vi "config UI.vi"() -> ()   [LabVIEW 2017, in "WaveformAcq editor node.lvclass"]
doc: "All child modules share this same UI. The UI allows for the configuration of Channels, Parameters, and Error Handling."
uses:
  WaveformAcq editor node.lvclass
  <vilib>/NI/Configuration Framework/Node/NodeRef.ctl
  <vilib>/NI/Configuration Framework/Node/NISE_CEF_Node.lvclass
  <vilib>/NI/AMC/Message Queue.ctl
  <vilib>/NI/AMC/Message.ctl
  <vilib>/NI/Tools/Keyed Array/KeyedArray.ctl
  <vilib>/NI/Configuration Framework/Node/UserEventRef.ctl
  <vilib>/NI/Configuration Framework/Controls/EventCluster.ctl
  <vilib>/NI/DCAF/Tag Editor Core/control module/configuration/error classification setting.ctl
  <vilib>/NI/Tag Bus Module Framework/runtime/error classification.ctl
  <vilib>/NI/Configuration Framework/Node/RefreshUIEvent.ctl
  <vilib>/NI/Configuration Framework/Node/CacheState.ctl
  <vilib>/NI/Configuration Framework/Node/StopEvent.ctl
  <vilib>/NI/Configuration Framework/Node/NodeChangeEvent.ctl
  <vilib>/NI/DCAF/Tag Editor Core/Table API/Available Tag Menu/channel action event.ctl
  <vilib>/NI/DCAF/Tag Editor Core/Table API/Available Tag Menu/dialog output action.ctl
  <vilib>/NI/Tag Bus Module Framework/channel/TBM channel.lvclass
  <vilib>/NI/Tag Bus/tag/tag descriptor.lvclass
  <vilib>/NI/DCAF/Tag Editor Core/Table API/Table Manager/Call Back Ref Type Def.ctl
  <vilib>/NI/DCAF/Tag Editor Core/Configuration Editor/Classes/Engine Parent/Engine Parent Editor Node.lvclass
  <vilib>/NI/DCAF/Tag Editor Core/Configuration Editor/Classes/Module editor node/module editor node.lvclass
  C:/Program Files (x86)/National Instruments/LabVIEW 2017/vi.lib/NI/Configuration Framework/serializable node/NISE_CEF_serializable node.lvclass
  <vilib>/NI/DCAF/Tag Editor Core/Table API/Table Manager/references.ctl
  <vilib>/NI/DCAF/Tag Editor Core/Table API/Table Manager/Menu Definition.ctl
  <vilib>/NI/DCAF/Tag Editor Core/Table API/Table Manager/Menu Options.ctl
  <vilib>/NI/DCAF/Tag Editor Core/control module/configuration/control module configuration.lvclass
  C:/Program Files (x86)/National Instruments/LabVIEW 2017/vi.lib/NI/Configuration Framework/serializable configuration/NISE_CEF_serializable configuration.lvclass
  module/configuration/WaveformAcq configuration.lvclass
  C:/Program Files (x86)/National Instruments/LabVIEW 2017/vi.lib/NI/DCAF/Tag Editor Core/control module/configuration/control module configuration.lvclass
  C:/Program Files (x86)/National Instruments/LabVIEW 2017/vi.lib/NI/Tag Bus Module Framework/module configuration/TBM module configuration.lvclass
  module/configuration/WaveformAcq configuration.lvclass/WaveformAcq configuration.ctl
  <vilib>/NI/DCAF/Tag Editor Core/control module/configuration/control module configuration.lvclass/control module configuration.ctl
  <vilib>/NI/Configuration Framework/serializable configuration/NISE_CEF_serializable configuration.lvclass/NISE_CEF_serializable configuration.ctl
  <vilib>/NI/Tag Bus Module Framework/channel/channel classification.ctl
  <vilib>/NI/DCAF/Tag Editor Core/control module/configuration/Write error classifications.vi
  <vilib>/NI/Tag Bus Module Framework/module configuration/TBM module configuration.lvclass
  <vilib>/NI/DCAF/Tag Editor Core/Configuration Editor/Classes/Module editor node/Read Module Configuration.vi
  <vilib>/Utility/LVClass/Get LV Class Name.vi
  <vilib>/NI/Configuration Framework/error generator/NISE_error generator.vi
  <vilib>/NI/DCAF/Tag Editor Core/Configuration Editor/Classes/Module editor node/Write Module Configuration.vi
  <vilib>/NI/Configuration Framework/serializable configuration/NISE_CEF_serializable configuration.lvclass
  <vilib>/NI/DCAF/Tag Editor Core/Table API/Listbox/Multi Column Listbox.lvclass
  <vilib>/NI/Configuration Framework/NISE_CEF_TreeControl.lvlib
  <vilib>/NI/DCAF/Tag Editor Core/Table API/Table Manager.lvlib
  <vilib>/NI/DCAF UI Toolkit/Controls/DCAF UI Elements.lvlib
  <vilib>/NI/Tools/Keyed Array/Tools_KeyedArray.lvlib
  <vilib>/NI/AMC/AMC.lvlib
  <vilib>/NI/DCAF/Tag Editor Core/Table API/Table Manager/Table Manager.lvclass
  <vilib>/NI/DCAF/Tag Editor Core/control module/editor node/control module editor.lvclass
  <vilib>/NI/Tag Bus Module Framework/runtime/TBM module execution interface.lvclass
panel:
  in  "Enum":i32
  in  "user event out":refnum<user-event>
  in  "Top Level Tab Control":T1(tab)
  in  "Channels Listbox":i32(listbox)
  in  "mapall":bool
  in  "mapwriters":bool
  in  "Parameters Listbox":i32(listbox)
  in  "Order":string[](array[string])
  in  "error classifications":T2[](array[typedef])
  in  "node change":T4
  in  "stop event":T5
  in  "cache state":T6
  in  "refresh UI":T7
  in  "user event":T8
  in  "main queue":T9
  in  "node ref":T10
  # "(Single-Click to Edit)"
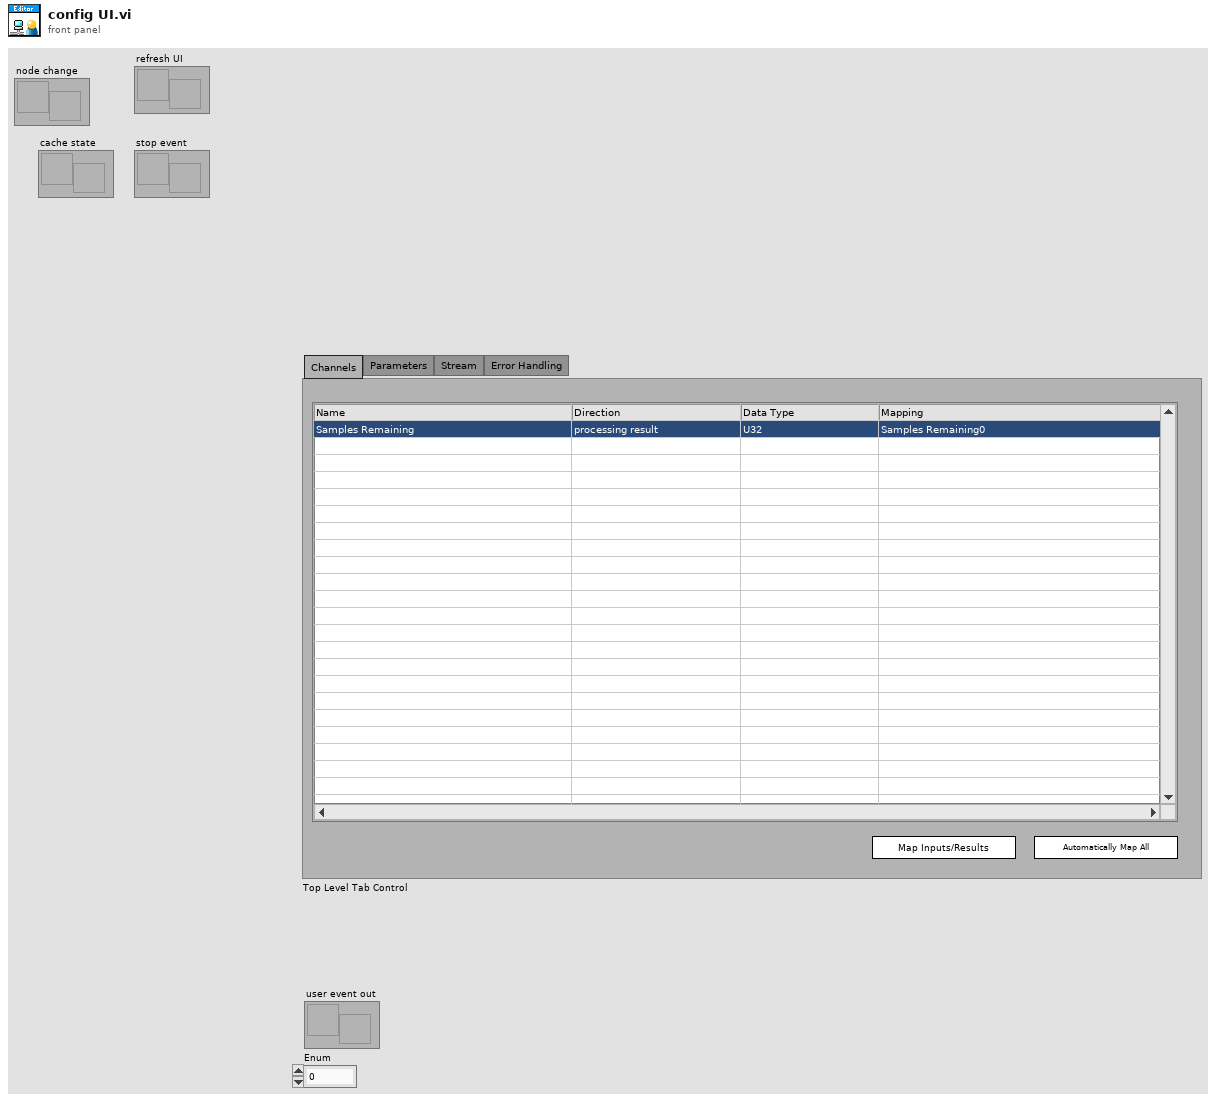
[diagram p1: front panel]
types:
  T1 = enum32{"Channels", "Parameters", "Stream", "Error Handling"}
  T2 = typedef "control module configuration.lvclass/error classification setting.ctl" = cluster{"code":i32, "error classification":T3}
  T3 = typedef "TBM module execution interface.lvclass/error classification.ctl" = enum16{"unknown", "none", "trivial", "recoverable", "critical"}
  T4 = typedef "NISE_CEF_Node.lvclass/NodeChangeEvent.ctl" = refnum<user-event>
  T5 = typedef "NISE_CEF_Node.lvclass/StopEvent.ctl" = refnum<user-event>
  T6 = typedef "NISE_CEF_Node.lvclass/CacheState.ctl" = refnum<user-event>
  T7 = typedef "NISE_CEF_Node.lvclass/RefreshUIEvent.ctl" = refnum<user-event>
  T8 = typedef "NISE_CEF_Node.lvclass/UserEventRef.ctl" = refnum<user-event>
  T9 = typedef "AMC.lvlib/Message Queue.ctl" = refnum<queue>
  T10 = typedef "NISE_CEF_Node.lvclass/NodeRef.ctl" = refnum<data-value>
  T11 = typedef "Table Manager.lvlib/Table Manager.lvclass/Menu Definition.ctl" = cluster{"Menu Name":string, "Menu Options":T12}
  T12 = typedef "Table Manager.lvlib/Table Manager.lvclass/Menu Options.ctl" = enum16{"Always Show", "Show When Used", "Show When Empty"}
  T13 = typedef "Table Manager.lvlib/Table Manager.lvclass/references.ctl" = cluster{"stop event":T5, "refresh UI":T7, "cache state":T6, "node change":T4, "user event out":refnum<user-event>, "main queue":T9, "user event":T8}
  T14 = typedef "Table Manager.lvlib/Column.lvclass/Column Descriptor.ctl" = cluster{"name":string, "caption":string, "Column Type":T15, "Params":string, "AutoSizeMode":i32, "FillWeight":sgl, "MinWidth":u32, "tooltip":string, "Enum Reference":refnum<vi>, "Channel suffix":string, "Read Only":bool, "Call Back VI":T16, "DT Dependency":i32, "name dependency":i32, "data type":T17, "Custom Column":refnum<class "Column.lvclass">}
  T15 = typedef "Table Manager.lvlib/Column.lvclass/Column Type.ctl" = enum16{"String", "Mapping", "Enum", "Custom"}
  T16 = typedef "Table Manager.lvlib/Table Manager.lvclass/Call Back Ref Type Def.ctl" = refnum<vi>
  T17 = typedef "tag bus.lvlib/tag descriptor.lvclass/Data Type.ctl" = enum16{"Double", "Single", "I64", "I32", "I16", "I8", "U64", "U32", "U16", "U8", "Boolean", "String", "Array of Double", "Array of Single", "Array of I64", "Array of I32", "Array of I16", "Array of I8", "Array of U64", "Array of U32", "Array of U16", "Array of U8", "Array of Boolean", "Array of String"}
  T18 = typedef "Table Manager.lvlib/Table Manager.lvclass/object ref.ctl" = cluster{"engine":refnum<data-value>, "Node Ref":refnum<data-value>}
  T19 = typedef "Table Manager.lvlib/Table Manager.lvclass/Table Events.ctl" = cluster{"Menu Selection":refnum<user-event>}
  T20 = typedef "NISE_CEF_TreeControl.lvlib/EventCluster.ctl" = cluster{"command":string, "data":string}
  T21 = typedef "TBM channel.lvclass/channel classification.ctl" = enum16{"input data", "output data", "processing parameter", "processing result"}
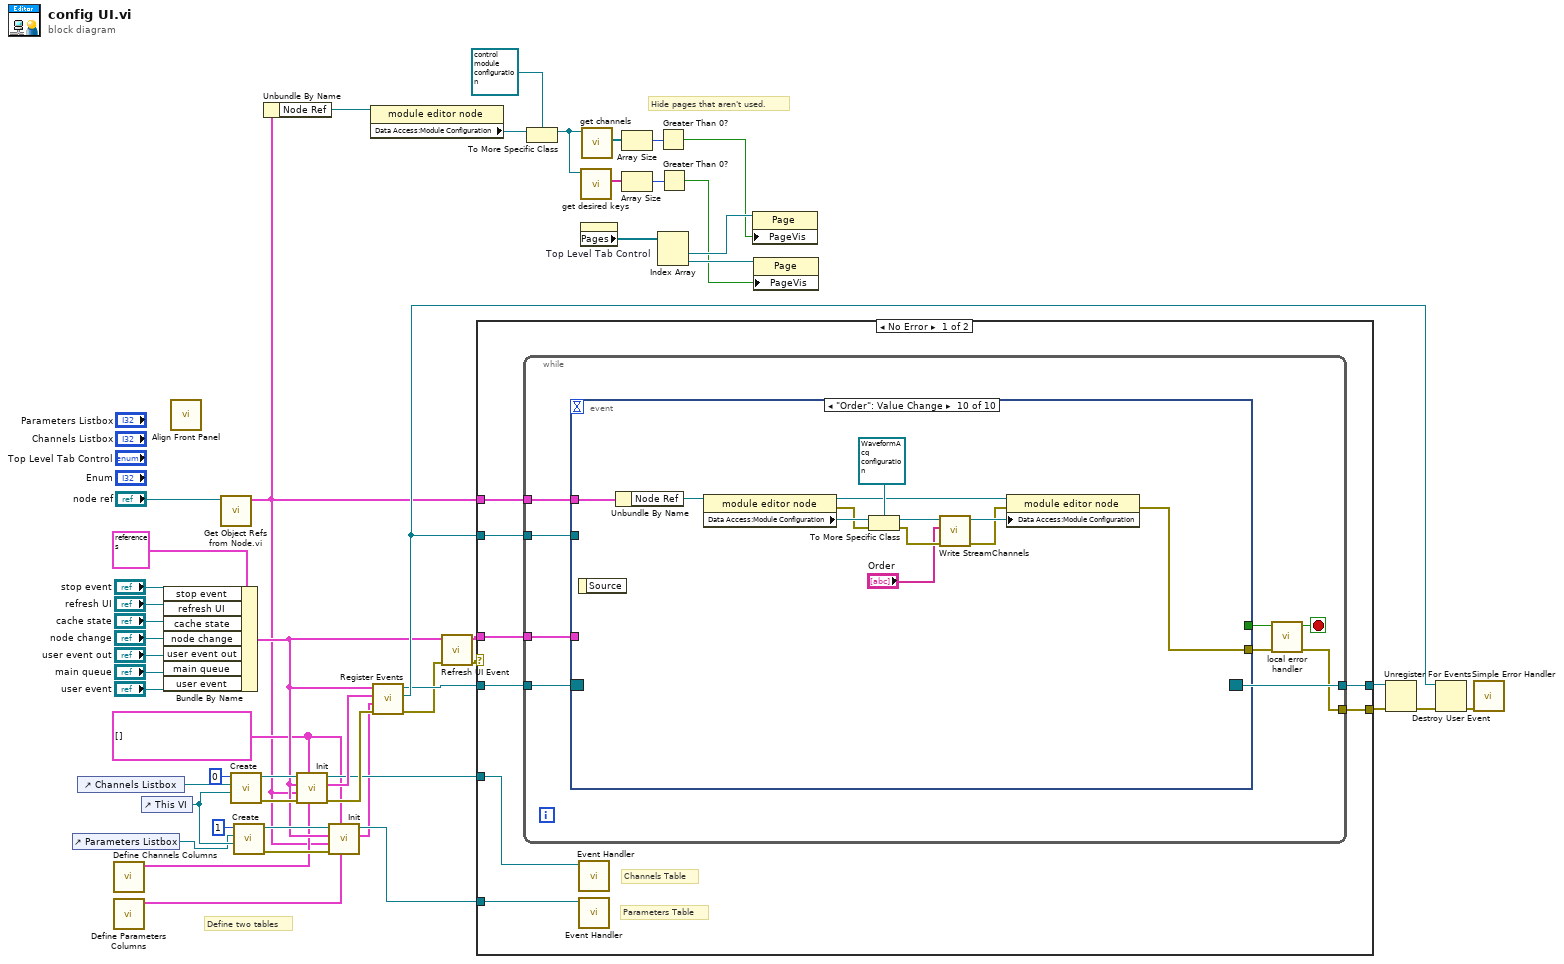
[diagram p0: block diagram]
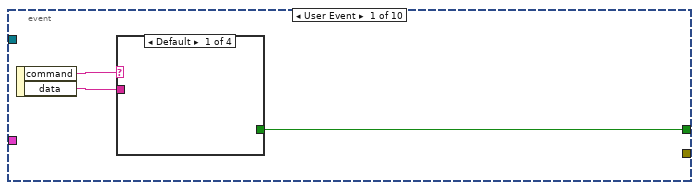
[diagram p2: hidden frame]
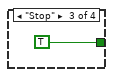
[diagram p4: hidden frame]
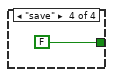
[diagram p5: hidden frame]
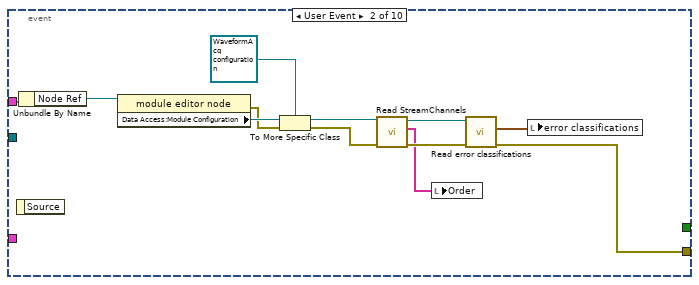
[diagram p6: hidden frame]
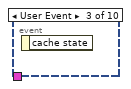
[diagram p7: hidden frame]
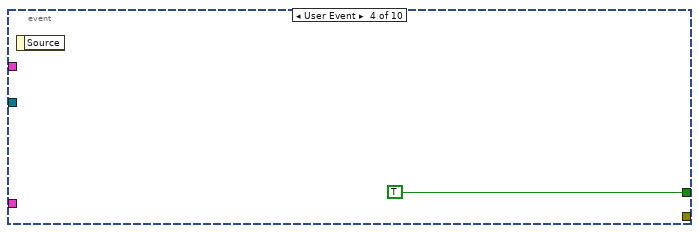
[diagram p8: hidden frame]
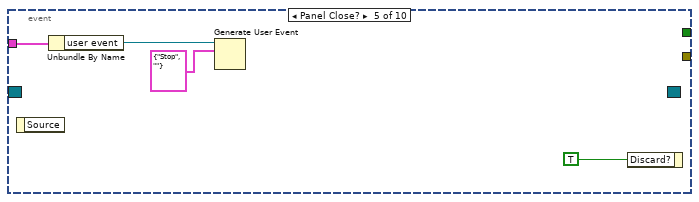
[diagram p9: hidden frame]
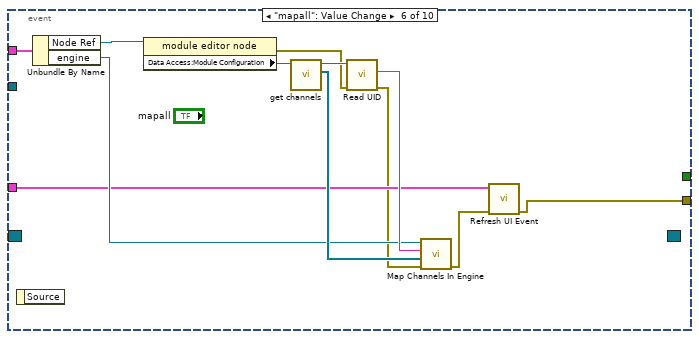
[diagram p10: hidden frame]
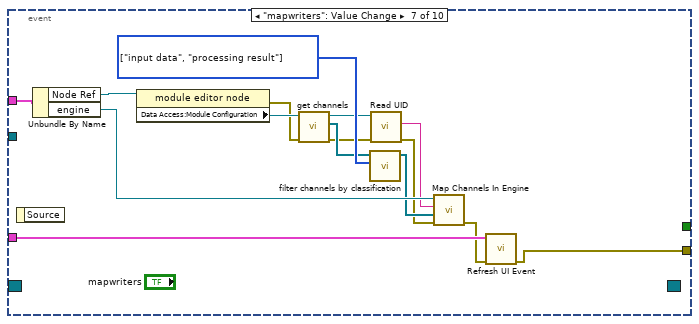
[diagram p11: hidden frame]
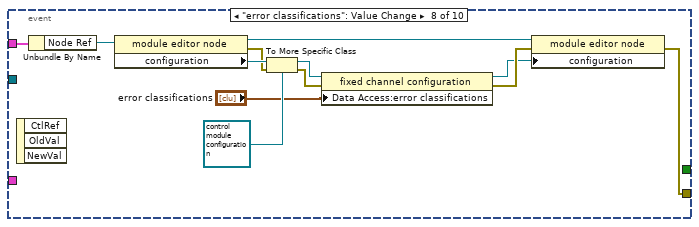
[diagram p12: hidden frame]
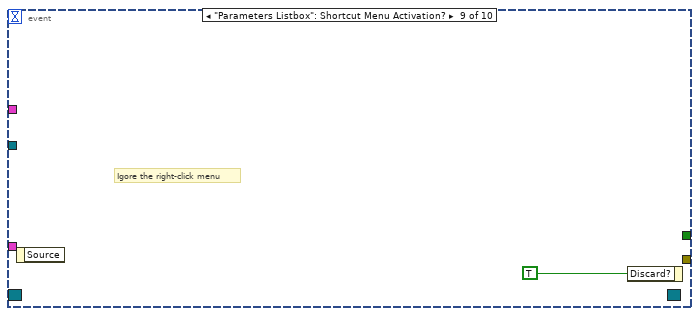
[diagram p13: hidden frame]
diagram:
  w15 = T11[] [] ("Right-Click Menu")
  # "Define two tables"
  # "Hide pages that aren't used."
  n1 = control-ref of="Parameters Listbox"() -> (w18:refnum<vi>)
  n2 = control-ref of="Channels Listbox"() -> (w26:refnum<vi>)
  n3 = call <vilib>:"Define Channels Columns.vi"() -> ("Column Descriptors"=w17:T14[])  [unwired: 11 in]
  n4 = call <vilib>:"Define Parameters Columns.vi"() -> ("Column Descriptors"=w16:T14[])  [unwired: 11 in]
  n5 = control-ref of="This VI"() -> (w22:refnum<vi>)
  n6 = Bundle By Name(cluster=T13 {"stop event"=refnum, "refresh UI"=refnum, "cache state"=refnum, "node change"=refnum, "user event out"=refnum, "main queue"=refnum, "user event"=refnum} ("Event References"), "stop event"="stop event", "refresh UI"="refresh UI", "cache state"="cache state", "node change"="node change", "user event out"="user event out", "main queue"="main queue", "user event"="user event") -> (w19:T13)
  n7 = call <vilib>:"Align Front Panel.vi"() -> ()  [unwired: 10 in, 2 out]
  n8 = call <vilib>:"Get Object Refs from Node.vi.vi"("node ref"="node ref") -> ("Node object refs"=w7:T18)  [unwired: 9 in, 1 out]
  n9 = call <vilib>:"Create.vi"("Top VI"=w22, "Listbox"=w26, "Index"=0) -> ("error out"=w29:errorcluster, "reference out"=w30:refnum<class "Multi Column Listbox.lvclass">)  [unwired: 7 in]
  n10 = call <vilib>:"Create.vi"("Top VI"=w22, "Listbox"=w18, "Index"=1) -> ("error out"=w25:errorcluster, "reference out"=w24:refnum<class "Multi Column Listbox.lvclass">)  [unwired: 7 in]
  n11 = Unbundle By Name(w7) -> ("Node Ref"=w5:refnum<data-value>)
  n12 = call-dynamic "Init.vi"("Column Descriptors"=w17, "Right-Click Menu"=w15, "error in (no error)"=w29, "Node object refs"=w7, "Event References"=w19, "Multi Column Listbox in"=w30) -> ("error out"=w28:errorcluster, "Table Events"=w40:T19, "Multi Column Listbox out"=w27:refnum<class "Multi Column Listbox.lvclass">)  [unwired: 3 in]
  n13 = call-dynamic "Init.vi"("Column Descriptors"=w16, "Right-Click Menu"=w15, "error in (no error)"=w25, "Node object refs"=w7, "Event References"=w19, "Multi Column Listbox in"=w24) -> ("Table Events"=w20:T19, "Multi Column Listbox out"=w21:refnum<class "Multi Column Listbox.lvclass">)  [unwired: 3 in, 1 out]
  n14 = property class="module editor node"(reference=w5) -> ("Data Access:Module Configuration"=w6:refnum<class "TBM module configuration.lvclass">)  [unwired: 1 in, 2 out]
  n15 = call <vilib>:"Register Events.vi"("error in (no error)"=w28, "Parameters Table Events"=w20, "Channels Table Events"=w40, "Event References"=w19) -> ("error out"=w33:errorcluster, "Channel Action"=w39:refnum<user-event>, "Event Registration Refnum"=w38:refnum<event-registration>)  [unwired: 5 in]
  n16 = call <vilib>:"Refresh UI Event.vi"("error in (no error)"=w33, "Event References"=w19) -> ("error out"=w34:errorcluster, "Event References out"=w32:T13)  [unwired: 8 in]
  n17 = case shown="No Error" w34 {
    selector: w34 -> [_ w142]
    tunnel: w38 -> [w58 w141]
    tunnel: [w57 w141] -> w50
    tunnel: [w55 w142] -> w49
    tunnel: w39 -> [w56 _]
    tunnel: w7 -> [w54 _]
    tunnel: w32 -> [w53 _]
    tunnel: w27 -> [w52 _]
    tunnel: w21 -> [w51 _]
    frame No Error {
      # "Parameters Table"
      # "Channels Table"
      n18 = while {
        tunnel: w58 -> [w67]
        tunnel: [w66] -> w57
        tunnel: w56 -> [w65]
        tunnel: [w61] -> w55
        tunnel: w54 -> [w60]
        tunnel: w53 -> [w59]
        stop <- w63 stop-if-true
        n19 = event shown="[9] \"Order\": Value Change" {
          selector: w67 -> [_ _ _ _ _ _ _ _ _ _]
          dyn-events: [_ _ _ _ _ _ _ _ _ _] -> w66
          timeout: _ -> [_ _ _ _ _ _ _ _ _ _]
          tunnel: [w70 _ _ TRUE _ _ _ _ _ _] -> w64
          tunnel: [_ w83 _ _ _ w95 w111 w127 _ w129] -> w62
          tunnel: w65 -> [_ _ _ _ _ _ _ _ _ _]
          tunnel: w60 -> [_ w84 _ _ _ w99 w112 w126 _ w140]
          tunnel: w59 -> [_ _ _ _ w87 w94 w110 _ _ _]
          event User Event {
            n20 = event-data() -> ("command"=w69:string, "data"=w68:string)  [unwired: 1 in]
            n21 = case shown="Default" w69 {
              tunnel: [_ _ TRUE FALSE] -> w70
              tunnel: w68 -> [_ _ _ _]
              frame Default {
              }
              frame "Refresh" {
              }
              frame "Stop" {
              }
              frame "save" {
              }
            }
          }
          event User Event {
            n22 = event-data() -> ()  [unwired: 1 in, 1 out]
            n23 = Unbundle By Name(w84) -> ("Node Ref"=w78:refnum<data-value>)
            n24 = property class="module editor node"(reference=w78) -> (error out=w74:errorcluster, "Data Access:Module Configuration"=w77:refnum<class "TBM module configuration.lvclass">)  [unwired: 1 in, 1 out]
            n25 = To More Specific Class(target class=refnum<class "WaveformAcq configuration.lvclass"> refnum ("WaveformAcq configuration in"), reference=w77, error in=w74) -> (specific class reference=w75:refnum<class "WaveformAcq configuration.lvclass">, error out=w73:errorcluster)
            n26 = call "Read StreamChannels.vi"("error in (no error)"=w73, "WaveformAcq configuration in"=w75) -> ("error out"=w80:errorcluster, "StreamChannels"=w79:string[], "WaveformAcq configuration out"=w81:refnum<class "WaveformAcq configuration.lvclass">)  [unwired: 7 in]
            n27 = local write "Order"(w79) -> ()
            n28 = call <vilib>:"Read error classifications.vi"("error in"=w80, "control module configuration in"=w81) -> ("error out"=w83:errorcluster, "error classifications"=w82:T2[])  [unwired: 7 in, 1 out]
            n29 = local write "error classifications"(w82) -> ()
          }
          event User Event {
            n30 = event-data() -> ()  [unwired: 1 in, 1 out]
          }
          event User Event {
            n31 = event-data() -> ()  [unwired: 1 in, 1 out]
          }
          event Panel Close? {
            n32 = event-data() -> ()  [unwired: 1 in, 1 out]
            n33 = Unbundle By Name(w87) -> ("user event"=w86:T8)
            n34 = Generate User Event(user event=w86, event data cluster=T20 {"command"="Stop", "data"=""} ("event data")) -> ()  [unwired: 2 in, 2 out]
            n35 = event-data("Discard?"=TRUE) -> ()  [unwired: 1 in, 1 out]
          }
          event "mapall": Value Change {
            n36 = event-data() -> ()  [unwired: 1 in, 1 out]
            n37 = Unbundle By Name(w99) -> ("Node Ref"=w98:refnum<data-value>, "engine"=w97:refnum<data-value>)
            n38 = property class="module editor node"(reference=w98) -> (error out=w91:errorcluster, "Data Access:Module Configuration"=w93:refnum<class "TBM module configuration.lvclass">)  [unwired: 1 in, 1 out]
            n39 = call-dynamic "get channels.vi"("module configuration in"=w93) -> ("channels"=w101:refnum<class "TBM channel.lvclass">[], "module configuration out"=w92:refnum<class "TBM module configuration.lvclass">)  [unwired: 9 in]
            n40 = call <vilib>:"Read UID.vi"("error in"=w91, "configuration in"=w92) -> ("error out"=w90:errorcluster, "instance id"=w100:string)  [unwired: 7 in, 1 out]
            n41 = call <vilib>:"Map Channels In Engine.vi"("error in (no error)"=w90, "channels"=w101, "instance id"=w100, "Engine DVR"=w97) -> ("error out"=w96:errorcluster)  [unwired: 7 in]
            n42 = call <vilib>:"Refresh UI Event.vi"("error in (no error)"=w96, "Event References"=w94) -> ("error out"=w95:errorcluster)  [unwired: 8 in, 1 out]
          }
          event "mapwriters": Value Change {
            w115 = T21[] [enum."input data", enum."processing result"] items=["input data", "output data", "processing parameter", "processing result"] ("allowed classifications")
            n43 = event-data() -> ()  [unwired: 1 in, 1 out]
            n44 = Unbundle By Name(w112) -> ("Node Ref"=w113:refnum<data-value>, "engine"=w109:refnum<data-value>)
            n45 = property class="module editor node"(reference=w113) -> (error out=w102:errorcluster, "Data Access:Module Configuration"=w104:refnum<class "TBM module configuration.lvclass">)  [unwired: 1 in, 1 out]
            n46 = call-dynamic "get channels.vi"("module configuration in"=w104) -> ("channels"=w114:refnum<class "TBM channel.lvclass">[], "module configuration out"=w103:refnum<class "TBM module configuration.lvclass">)  [unwired: 9 in]
            n47 = call <vilib>:"filter channels by classification.vi"("allowed classifications"=w115, "channels in"=w114) -> ("channels out"=w107:refnum<class "TBM channel.lvclass">[])  [unwired: 9 in]
            n48 = call <vilib>:"Read UID.vi"("error in"=w102, "configuration in"=w103) -> ("error out"=w106:errorcluster, "instance id"=w108:string)  [unwired: 7 in, 1 out]
            n49 = call <vilib>:"Map Channels In Engine.vi"("error in (no error)"=w106, "channels"=w107, "instance id"=w108, "Engine DVR"=w109) -> ("error out"=w105:errorcluster)  [unwired: 7 in]
            n50 = call <vilib>:"Refresh UI Event.vi"("error in (no error)"=w105, "Event References"=w110) -> ("error out"=w111:errorcluster)  [unwired: 8 in, 1 out]
          }
          event "error classifications": Value Change {
            n51 = event-data() -> ()  [unwired: 1 in, 3 out]
            n52 = Unbundle By Name(w126) -> ("Node Ref"=w121:refnum<data-value>)
            n53 = property class="module editor node"(reference=w121) -> (reference out=w125:refnum<data-value>, error out=w117:errorcluster, "configuration"=w120:refnum<class "NISE_CEF_serializable configuration.lvclass">)  [unwired: 1 in]
            n54 = To More Specific Class(target class=refnum<class "control module configuration.lvclass"> refnum ("fixed channel configuration"), reference=w120, error in=w117) -> (specific class reference=w122:refnum<class "control module configuration.lvclass">, error out=w116:errorcluster)
            n55 = property class="fixed channel configuration"(reference=w122, error in=w116, "Data Access:error classifications"="error classifications") -> (reference out=w123:refnum<class "control module configuration.lvclass">, error out=w124:errorcluster)
            n56 = property class="module editor node"(reference=w125, error in=w124, "configuration"=w123) -> (error out=w127:errorcluster)  [unwired: 1 out]
          }
          event "Parameters Listbox": Shortcut Menu Activation? {
            # "Igore the right-click menu"
            n57 = event-data() -> ()  [unwired: 1 in, 1 out]
            n58 = event-data("Discard?"=TRUE) -> ()  [unwired: 1 in, 1 out]
          }
          event "Order": Value Change {
            n59 = event-data() -> ()  [unwired: 1 in, 1 out]
            n60 = Unbundle By Name(w140) -> ("Node Ref"=w139:refnum<data-value>)
            n61 = property class="module editor node"(reference=w139) -> (reference out=w132:refnum<data-value>, error out=w137:errorcluster, "Data Access:Module Configuration"=w138:refnum<class "TBM module configuration.lvclass">)  [unwired: 1 in]
            n62 = To More Specific Class(target class=refnum<class "WaveformAcq configuration.lvclass"> refnum ("WaveformAcq configuration"), reference=w138, error in=w137) -> (specific class reference=w136:refnum<class "WaveformAcq configuration.lvclass">, error out=w134:errorcluster)
            n63 = call "Write StreamChannels.vi"("error in (no error)"=w134, "StreamChannels"="Order", "WaveformAcq configuration in"=w136) -> ("error out"=w130:errorcluster, "WaveformAcq configuration out"=w131:refnum<class "WaveformAcq configuration.lvclass">)  [unwired: 7 in]
            n64 = property class="module editor node"(reference=w132, error in=w130, "Data Access:Module Configuration"=w131) -> (error out=w129:errorcluster)  [unwired: 1 out]
          }
        }
        n65 = call <vilib>:"local error handler.vi"("error in (no error)"=w62, "Stop in"=w64) -> ("error out"=w61:errorcluster, "Stop out"=w63:bool)  [unwired: 8 in]
      }
      n66 = call-dynamic "Event Handler.vi"("Listbox in"=w52) -> ()  [unwired: 9 in, 2 out]
      n67 = call-dynamic "Event Handler.vi"("Listbox in"=w51) -> ()  [unwired: 9 in, 2 out]
    }
    frame Error {
    }
  }
  n68 = To More Specific Class(target class=refnum<class "control module configuration.lvclass"> refnum ("fixed channel configuration"), reference=w6) -> (specific class reference=w3:refnum<class "control module configuration.lvclass">)  [unwired: 1 in, 1 out]
  n69 = call-dynamic "get desired keys.vi"("fixed channel configuration in"=w3) -> ("desired keys"=w11:string[])  [unwired: 8 in, 2 out]
  n70 = property on="Top Level Tab Control" class="TabCtl (strict)"() -> ("Pages"=w8:refnum<vi>[])  [unwired: 2 in, 2 out]
  n71 = call-dynamic "get channels.vi"("fixed channel configuration in"=w3) -> ("channels"=w14:refnum<class "TBM channel.lvclass">[])  [unwired: 9 in, 1 out]
  n72 = Array Size(array=w14) -> (size(s)=w13:i32)
  n73 = Array Size(array=w11) -> (size(s)=w12:i32)
  n74 = Greater Than 0?(x=w13) -> (x > 0?=w2:bool)
  n75 = Index Array(array=w8) -> (element #1=w9:refnum<vi>, element #2=w10:refnum<vi>)  [unwired: 2 in]
  n76 = Greater Than 0?(x=w12) -> (x > 0?=w1:bool)
  n77 = property class="Page"(reference=w9, "PageVis"=w2) -> ()  [unwired: 1 in, 2 out]
  n78 = property class="Page"(reference=w10, "PageVis"=w1) -> ()  [unwired: 1 in, 2 out]
  n79 = Unregister For Events(event registration refnum=w50, error in=w49) -> (error out=w48:errorcluster)
  n80 = Destroy User Event(user event=w39, error in=w48) -> (error out=w47:errorcluster)
  n81 = call <vilib>:"Simple Error Handler.vi"("error in (no error)"=w47) -> ()  [unwired: 4 in, 5 out]
